vi "TimeInterval.vi"(11 "Time Interval":dbl format="%.6f") -> (3 "Time interval in Hex":u32 format="%x")   [LabVIEW 2016]
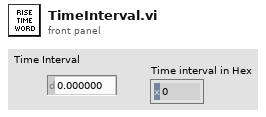
[diagram p1: front panel]
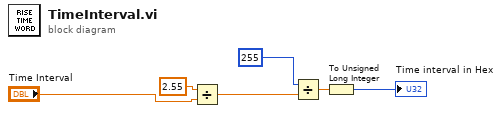
[diagram p0: block diagram]
diagram:
  n1 = Divide(x=2.55, y="Time Interval") -> (x/y=w3:dbl)
  n2 = Divide(x=u32 255, y=w3) -> (x/y=w4:dbl)
  n3 = To Unsigned Long Integer(number=w4) -> (unsigned 32bit integer=→"Time interval in Hex":u32)
